vi "TwReadRawDataLV.vi"() -> ()   [LabVIEW 2009]
panel:
  out "buffer out":u8[](array[numeric])
  out "error out":errorcluster
  in  "error in (no error)":errorcluster
  in  "writeIndex":i32
  in  "bufIndex":i32
  in  "channel":i32
  in  "filename":string
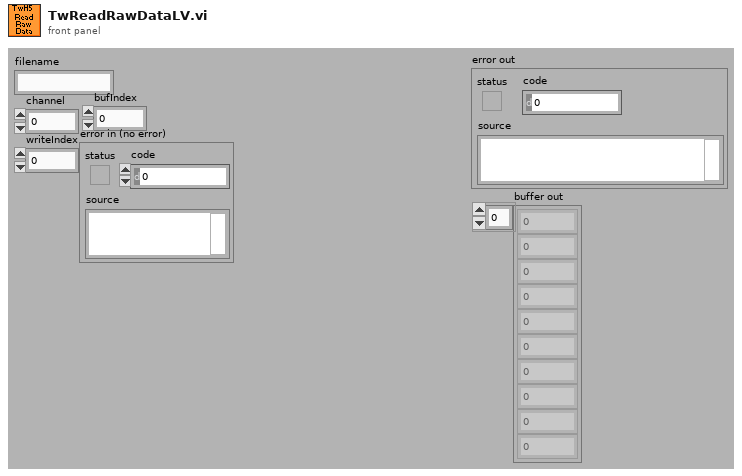
[diagram p1: front panel]
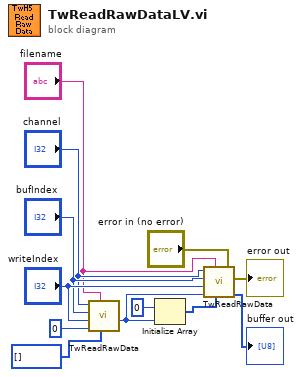
[diagram p0: block diagram]
diagram:
  n1 = call "TwReadRawData.vi"("buffer"=u8[] [], "filename"="filename", "bufferSize in"=0, "writeIndex"="writeIndex", "bufIndex"="bufIndex", "channel"="channel") -> ("bufferSize out"=w8:i32)  [unwired: 1 in, 2 out]
  n2 = Initialize Array(u8 0 ("element"), w8) -> (w9:u8[])
  n3 = call "TwReadRawData.vi"("error in (no error)"="error in (no error)", "buffer"=w9, "filename"="filename", "bufferSize in"=w8, "writeIndex"="writeIndex", "bufIndex"="bufIndex", "channel"="channel") -> ("buffer out"=→"buffer out":u8[], "error out"=→"error out":errorcluster)  [unwired: 1 out]
